vi "Version.vi"(8 "error in (no error)":errorcluster, 11 "MicronCLI in":refnum<class "MicronCLI.lvclass">) -> (0 "error out":errorcluster, 2 "Version":string, 3 "MicronCLI out":refnum<class "MicronCLI.lvclass">)   [LabVIEW 2019, in "MicronCLI.lvclass"]
uses:
  MicronCLI.lvclass
  MicronCLI.lvclass/MicronCLI.ctl
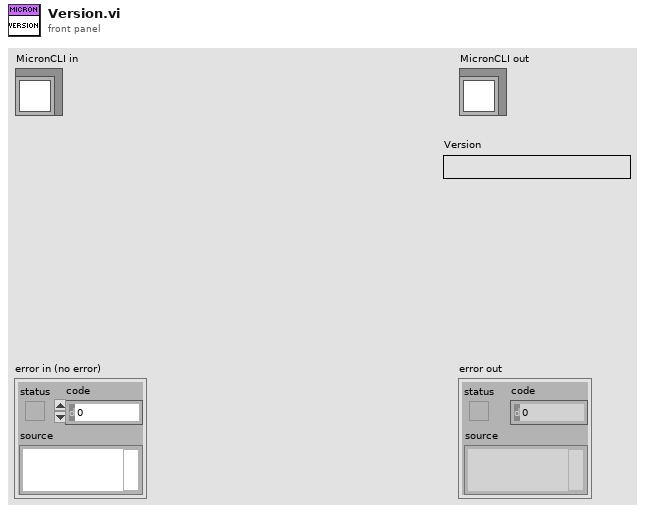
[diagram p1: front panel]
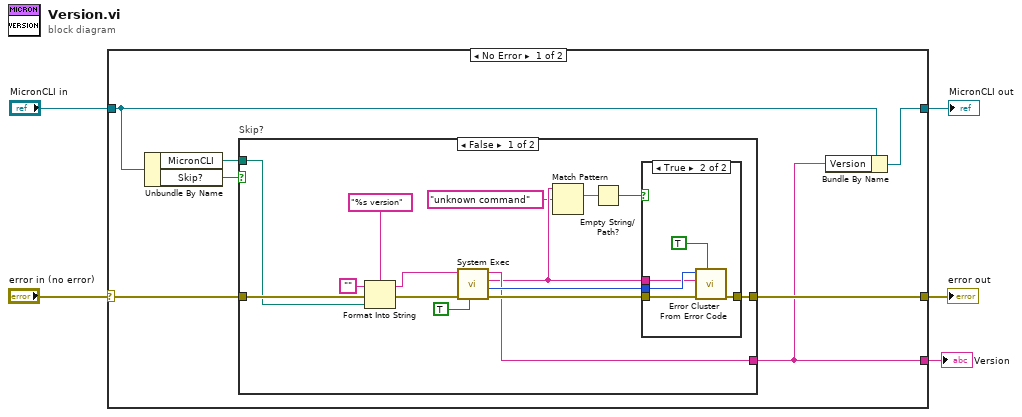
[diagram p0: block diagram]
diagram:
  n1 = case shown="No Error" "error in (no error)" {
    selector: "error in (no error)" -> [w12 w36]
    tunnel: [w10 w36] -> w4
    tunnel: [w7 w35] -> w2
    tunnel: "MicronCLI in" -> [w8 w35]
    tunnel: [w6 _] -> w1
    frame No Error {
      n2 = Unbundle By Name(w8) -> ("MicronCLI"=w11:path, "Skip?"=w9:bool)
      n3 = case "Skip?" shown="False" w9 {
        tunnel: w12 -> [w27 w34]
        tunnel: w11 -> [w23 _]
        tunnel: [w19 w34] -> w10
        tunnel: [w17 _] -> w6
        frame False {
          n4 = Format Into String(format string="%s version", initial string="", error in=w27, w23) -> (resulting string=w21:string, error out=w25:errorcluster)
          n5 = call <vilib>:"System Exec.vi"("run minimized? (F)"=TRUE, "error in (no error)"=w25, "command line"=w21) -> ("error out"=w26:errorcluster, "return code"=w18:i32, "standard error"=w16:string, "standard output"=w17:string)  [unwired: 5 in]
          n6 = Match Pattern(string=w16, regular expression="unknown command") -> (match substring=w14:string)  [unwired: 1 in, 3 out]
          n7 = Empty String/Path?(string/path=w14) -> (empty?=w13:bool)
          n8 = case shown="True" w13 {
            tunnel: w26 -> [w28 w33]
            tunnel: [w28 w32] -> w19
            tunnel: w18 -> [_ w31]
            tunnel: w16 -> [_ w29]
            frame False {
              # "Ignore if version command is not present"
            }
            frame True {
              n9 = call <vilib>:"Error Cluster From Error Code.vi"("show call chain? (False)"=TRUE, "error in (no error)"=w33, "error message (\"\")"=w29, "error code (0)"=w31) -> ("error out"=w32:errorcluster)  [unwired: 5 in]
            }
          }
        }
        frame True {
        }
      }
      n10 = Bundle By Name(cluster=w8, "Version"=w6) -> (w7:refnum<class "MicronCLI.lvclass">)
    }
    frame Error {
    }
  }
  "error out" <- w4
  "MicronCLI out" <- w2
  "Version" <- w1
